vi "DSF.Engine.Transfer Group.Get Return FIFO.vi"(11 "Transfer Group in":refnum<class "DSF.Engine.Transfer Group.lvclass">) -> (2 "Return FIFO":refnum<k33>, 3 "Transfer Group out":refnum<class "DSF.Engine.Transfer Group.lvclass">)   [LabVIEW 2017, in "DSF.Engine.lvlib" / "DSF.Engine.Transfer Group.lvclass"]
uses:
  DSF.Engine.Transfer Group.lvclass
  DSF.Engine.Transfer Group.lvclass/DSF.Engine.Transfer Group.ctl
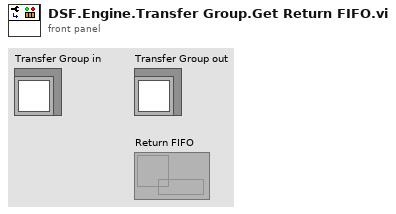
[diagram p1: front panel]
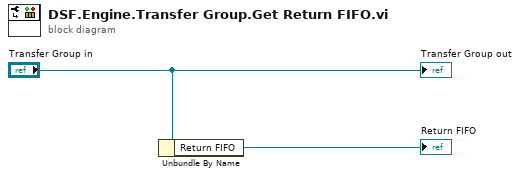
[diagram p0: block diagram]
diagram:
  n1 = Unbundle By Name("Transfer Group in") -> ("Return FIFO"=→"Return FIFO":refnum<k33>)
  "Transfer Group out" <- "Transfer Group in"
